vi "Page_Source_Remove.vi"(4 "sourceInclusion":T1, 6 "ctlReferences":T2, 7 "Project Refnum":refnum<vi>, 8 "error in (no error)":errorcluster, 9 "bottomTree?":bool, 10 "disableSource":bool, 11 "AB_Source_Library in":refnum<class "AB_Source_Library.lvclass">) -> (0 "error out":errorcluster, 3 "AB_Source_Library out":refnum<class "AB_Source_Library.lvclass">)   [LabVIEW 2020, in "AB_Source_Library.lvclass"]
uses:
  <vilib>/AppBuilder/AB_Classes/Source/Library/AB_Source_Library.lvclass
  e:/builds/penguin/labview/branches/2020/dev/dist/vi.lib/AppBuilder/AB_Classes/Source/AB_Source.lvclass
  <resource>/Framework/Providers/Builds/AppBuilder/AB_UI_Page_Source_Files_References.ctl
  <vilib>/AppBuilder/AB_Source_Inclusion.ctl
  <vilib>/AppBuilder/AB_Classes/Source/Library/AB_Source_Library.lvclass/AB_Source_Library.ctl
  <vilib>/AppBuilder/AB_Classes/Source/AB_Source.lvclass
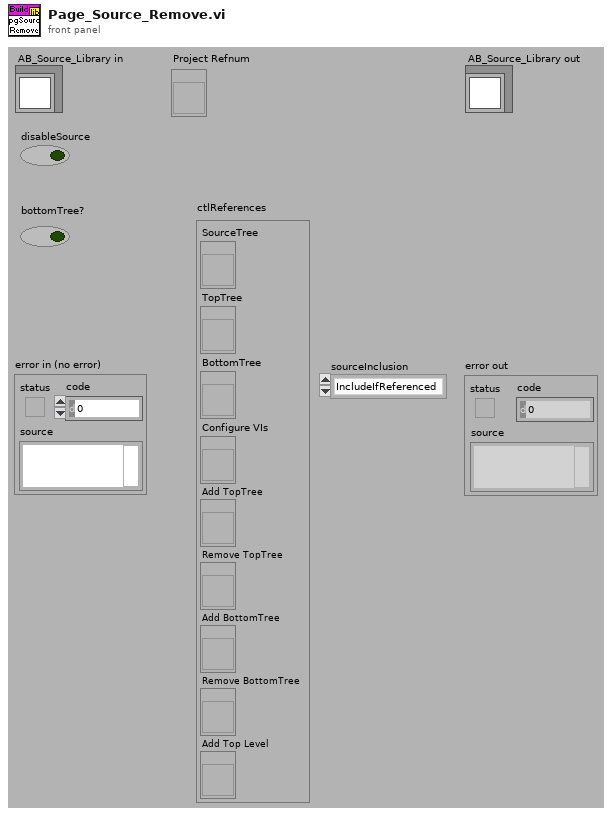
[diagram p1: front panel]
types:
  T1 = typedef "AB_Source_Inclusion.ctl" = enum16{"IncludeIfReferenced", "Include", "Exclude", "TopLevel"}
  T2 = typedef "AB_UI_Page_Source_Files_References.ctl" = cluster{"SourceTree":refnum<vi>, "TopTree":refnum<vi>, "BottomTree":refnum<vi>, "Configure VIs":refnum<vi>, "Add TopTree":refnum<vi>, "Remove TopTree":refnum<vi>, "Add BottomTree":refnum<vi>, "Remove BottomTree":refnum<vi>, "Add Top Level":refnum<vi>}
  T3 = typedef "AB_Source.ctl" = cluster{"path":path, "itemID":string, "parentIndex":i32, "sourceInclusion":T1, "destinationIndex":i32, "properties":T4[], "newName":string, "lvfile":bool, "valid":bool, "eng_inBuild":bool, "eng_isNonVILink":bool, "Amalgamation":bool, "Amalgamation Piece":bool, "eng_delimitedName":string, "preventRename":bool}
  T4 = typedef "AB_Source_Properties.ctl" = cluster{"sourcePropertyType":T5, "value":variant}
  T5 = typedef "AB_Source_Property_Type.ctl" = enum16{"Remove block diagram", "Remove front panel", "Password", "Window has title bar", "Show menu bar", "Show vertical scroll bar", "Show horizontal scroll bar", "Show toolbar", "Show Abort button", "Show fp when called", "Window behavior", "Allow user to close window", "Window run-time position", "Run when opened", "Allow debugging", "Auto error handling", "Generate guard code", "Use stack variables", "Expression folding", "Integer only", "Inline subVI"}
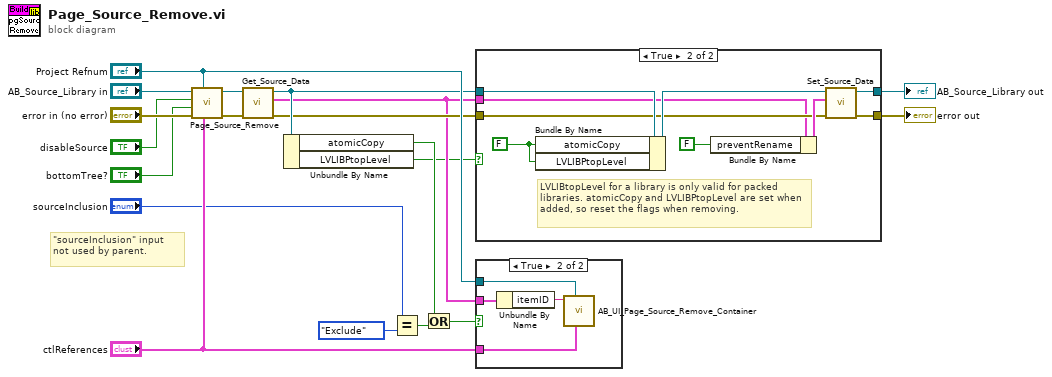
[diagram p0: block diagram]
diagram:
  # "\"sourceInclusion\" input not used by parent."
  n1 = call-parent "Page_Source_Remove.vi"("ctlReferences"="ctlReferences", "Project Refnum"="Project Refnum", "error in (no error)"="error in (no error)", "bottomTree?"="bottomTree?", "disableSource"="disableSource", "AB_Source in"="AB_Source_Library in") -> ("error out"=w15:errorcluster, "AB_Source out"=w16:refnum<class "AB_Source_Library.lvclass">)  [unwired: 4 in]
  n2 = call <vilib>:"Get_Source_Data.vi"("error in (no error)"=w15, "Class in"=w16) -> ("error out"=w4:errorcluster, "data"=w2:T3, "Class out"=w6:refnum<class "AB_Source_Library.lvclass">)  [unwired: 7 in]
  n3 = Unbundle By Name(w6) -> ("atomicCopy"=w12:bool, "LVLIBPtopLevel"=w1:bool)
  n4 = Equal?(x="sourceInclusion", y=AB_Source_Inclusion."Exclude") -> (x = y?=w11:bool)
  n5 = Or(x=w12, y=w11) -> (x .or. y?=w9:bool)
  n6 = case shown="True" w1 {
    tunnel: w6 -> [w21 w30]
    tunnel: [w21 w26] -> w5
    tunnel: w4 -> [w20 w24]
    tunnel: [w20 w23] -> w3
    tunnel: w2 -> [_ w22]
    frame False {
    }
    frame True {
      w29 = FALSE ("data.atomicCopy")
      # "LVLIBtopLevel for a library is only valid for packed libraries. atomicCopy and LVLIBPtopLevel are set when added, so reset the flags when removing."
      n7 = Bundle By Name(cluster=w30, "atomicCopy"=w29, "LVLIBPtopLevel"=w29) -> (w25:refnum<class "AB_Source_Library.lvclass">)
      n8 = Bundle By Name(cluster=w22, "preventRename"=FALSE) -> (w27:T3)
      n9 = call <vilib>:"Set_Source_Data.vi"("error in (no error)"=w24, "data"=w27, "Class in"=w25) -> ("error out"=w23:errorcluster, "Class out"=w26:refnum<class "AB_Source_Library.lvclass">)  [unwired: 7 in]
    }
  }
  "error out" <- w3
  "AB_Source_Library out" <- w5
  n10 = case shown="True" w9 {
    tunnel: w2 -> [_ w33]
    tunnel: "ctlReferences" -> [_ w32]
    tunnel: "Project Refnum" -> [_ w31]
    frame False {
    }
    frame True {
      n11 = Unbundle By Name(w33) -> ("itemID"=w34:string)
      n12 = call <resource>:"AB_UI_Page_Source_Remove_Container.vi"("ctlReferences"=w32, "Project Refnum"=w31, "itemID"=w34) -> ()  [unwired: 8 in, 1 out]
    }
  }
